vi "TDMS2TDMLogIllegalName.vi"(8 "error in (no error)":errorcluster, 10 "New Name":string, 11 "Original Name":string) -> (0 "error out":errorcluster)   [LabVIEW 2017]
doc: "This VI reports in the log text that an illegal name has been coerced to a name that fits the TDM storage format."
uses:
  <vilib>/Utility/tdmsutil.llb/TDMS2TDMLogOperation.ctl
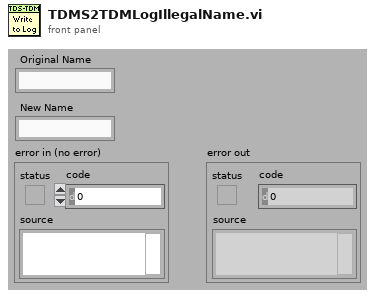
[diagram p1: front panel]
types:
  T1 = typedef "TDMS2TDMLogOperation.ctl" = enum16{"Initialize", "Data Conversion", "Name Conversion", "Write Log File"}
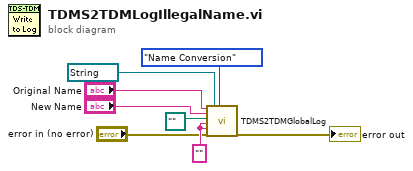
[diagram p0: block diagram]
diagram:
  w6 = "" ("Original Name")
  n1 = call <vilib>:"TDMS2TDMGlobalLog.vi"("Original Name"="Original Name", "New Name"="New Name", "Log File Path"=path "", "Original Datatype"=w6, "New Datatype"=w6, "error in (no error)"="error in (no error)", "Str Refnum"=refnum<vi> refnum, "Operation"=TDMS2TDMLogOperation."Name Conversion") -> ("error out"=→"error out":errorcluster)  [unwired: 11 in]
